vi "DriveModuleTrend.vi"(11 "Module":i32) -> ()   [LabVIEW 2023]
uses:
  <vilib>/Rock Robotics/Network Tables/NT Read Number.vi
  <vilib>/Rock Robotics/Network Tables/NT Read Boolean.vi
panel:
  out "Const":bool
  out "Plant":bool
  out "PID_Done":bool
  out "CoStdDev":dbl format="%_8e"
  out "PvStdDev":dbl format="%_8e"
  out "Kd":dbl format="%_8e"
  out "Ki":dbl format="%_8e"
  out "Kp":dbl format="%_8e"
  out "Ka_StdDev":dbl format="%_8e"
  out "Ka_Calc":dbl format="%_8e"
  out "Ka_Done":bool
  out "Kv_SlowBck":dbl format="%_8e"
  out "Kv_SlowFwd":dbl format="%_8e"
  out "Kv_FastFwd":dbl format="%_8e"
  out "Swerve Mod":i32 format="%11.0f"
  out "Waveform Chart":T1(graph)
  out "Abs Angle Deg":dbl format="%11.1f"
  out "Dist Ft":dbl format="%11.2f"
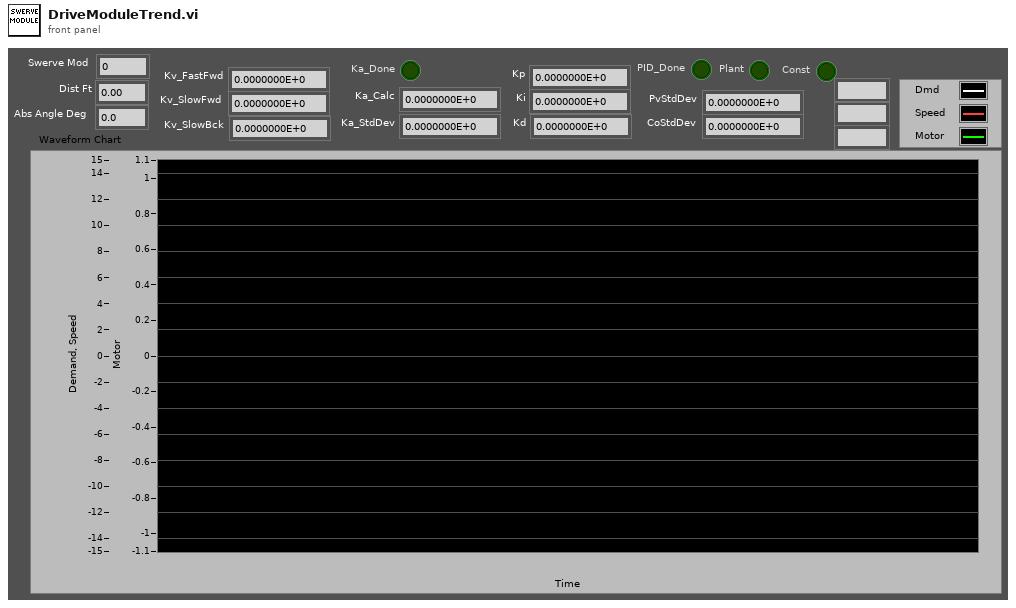
[diagram p1: front panel]
types:
  T1 = cluster{"TravSpdDmdFPS":dbl, "TravSpeedFPS":dbl, "TravMotDmd":dbl}
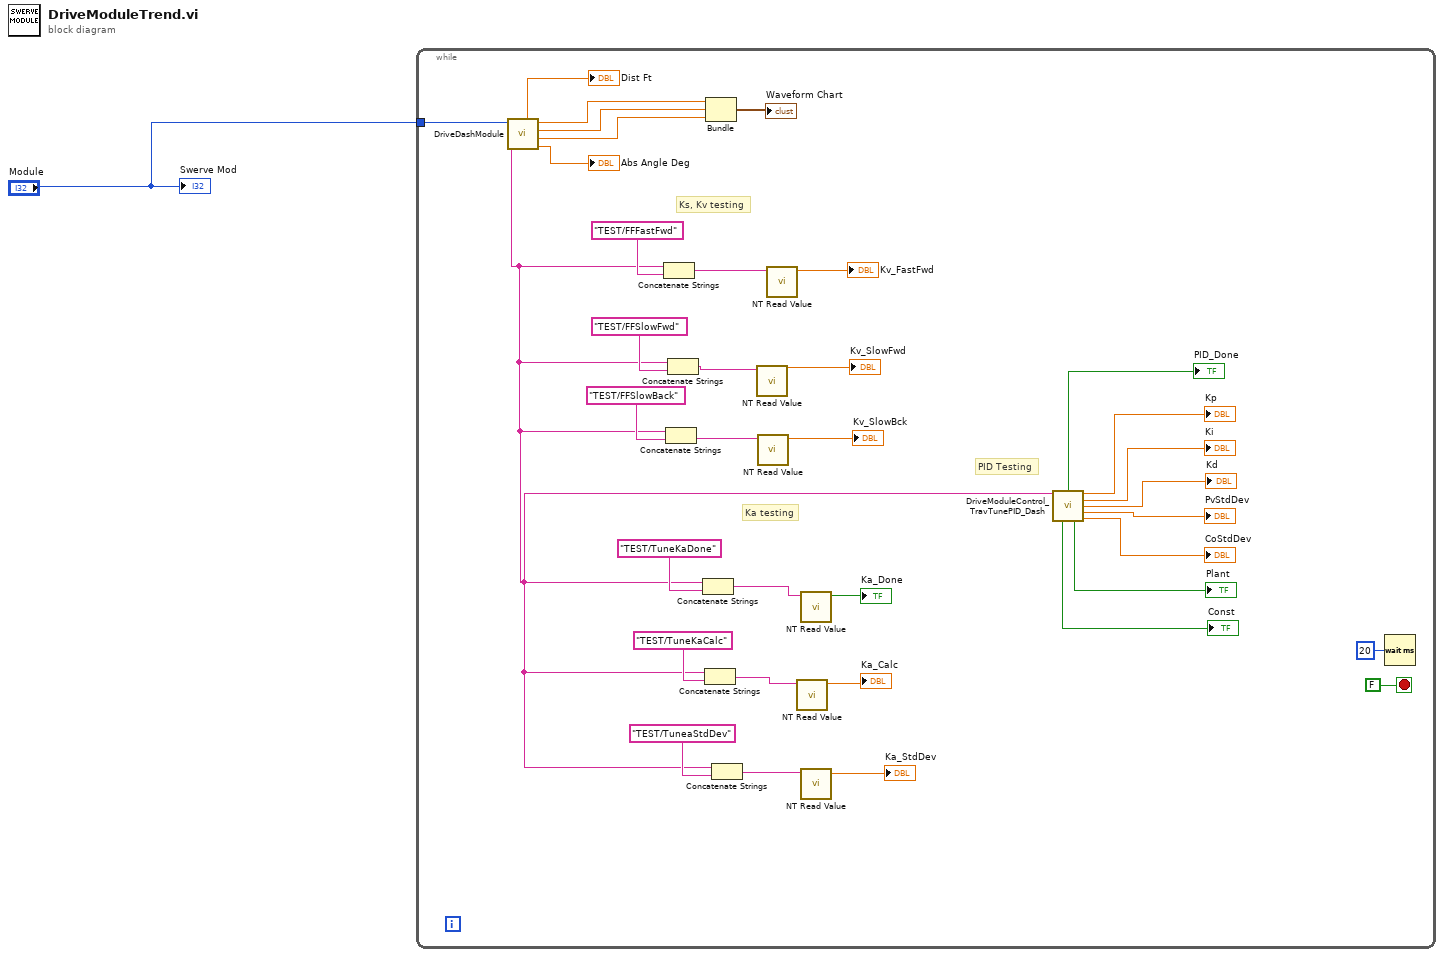
[diagram p0: block diagram]
diagram:
  n1 = while {
    tunnel: "Module" -> [w35]
    stop <- FALSE stop-if-true
    # "PID Testing"
    # "Ka testing"
    # "Ks, Kv testing"
    n2 = call "DriveDashModule.vi"("Module"=w35) -> ("SpinAbsPosDeg"=→"Abs Angle Deg":dbl, "TravMotDmd"=w32:dbl, "TravSpeedFPS"=w33:dbl, "TravSpdDmdFPS"=w34:dbl, "TravDistFt"=→"Dist Ft":dbl, "Prefix"=w10:string)  [unwired: 5 in]
    n3 = Concatenate Strings(w10, "TEST/FFFastFwd" ("refnum name")) -> (w27:string)
    n4 = Concatenate Strings(w10, "TEST/FFSlowBack" ("refnum name")) -> (w23:string)
    n5 = Concatenate Strings(w10, "TEST/FFSlowFwd" ("refnum name")) -> (w24:string)
    n6 = Concatenate Strings(w10, "TEST/TuneKaDone" ("name")) -> (w16:string)
    n7 = Concatenate Strings(w10, "TEST/TuneKaCalc" ("name")) -> (w15:string)
    n8 = Bundle("TravSpdDmdFPS"=w34, "TravSpeedFPS"=w33, "TravMotDmd"=w32) -> (→"Waveform Chart":T1)  [unwired: 1 in]
    n9 = Concatenate Strings(w10, "TEST/TuneaStdDev" ("name")) -> (w14:string)
    n10 = call-poly <vilib>:"NT Read Value.vi"("name"=w24) -> ("value"=→"Kv_SlowFwd":dbl)  [unwired: 8 in, 2 out]
    n11 = call-poly <vilib>:"NT Read Value.vi"("name"=w23) -> ("value"=→"Kv_SlowBck":dbl)  [unwired: 8 in, 2 out]
    n12 = call-poly <vilib>:"NT Read Value.vi"("name"=w27) -> ("value"=→"Kv_FastFwd":dbl)  [unwired: 8 in, 2 out]
    n13 = call-poly <vilib>:"NT Read Value.vi"("name"=w15) -> ("value"=→"Ka_Calc":dbl)  [unwired: 8 in, 2 out]
    n14 = call-poly <vilib>:"NT Read Value.vi"("name"=w16) -> ("value"=→"Ka_Done":bool)  [unwired: 8 in, 2 out]
    n15 = call-poly <vilib>:"NT Read Value.vi"("name"=w14) -> ("value"=→"Ka_StdDev":dbl)  [unwired: 8 in, 2 out]
    n16 = call "DriveModuleControl_TravTunePID_Dash.vi"("Network Table Prefix"=w10) -> ("TestDone"=→"PID_Done":bool, "Kp"=→"Kp":dbl, "Ki"=→"Ki":dbl, "Kd"=→"Kd":dbl, "PvStdDev"=→"PvStdDev":dbl, "ConstDone"=→"Const":bool, "PlantDone"=→"Plant":bool, "CoStdDev"=→"CoStdDev":dbl)  [unwired: 5 in, 2 out]
    n17 = Wait (ms)(milliseconds to wait=u32 20) -> ()  [unwired: 1 out]
  }
  "Swerve Mod" <- "Module"
